vi "ReadMJPEGStream.vi"(11 "url":string="http://localhost:8000") -> (0 "error out":errorcluster, 2 "Info":T1, 3 "TCP out":refnum<k5>)   [LabVIEW 2020]
panel:
  out "path":string
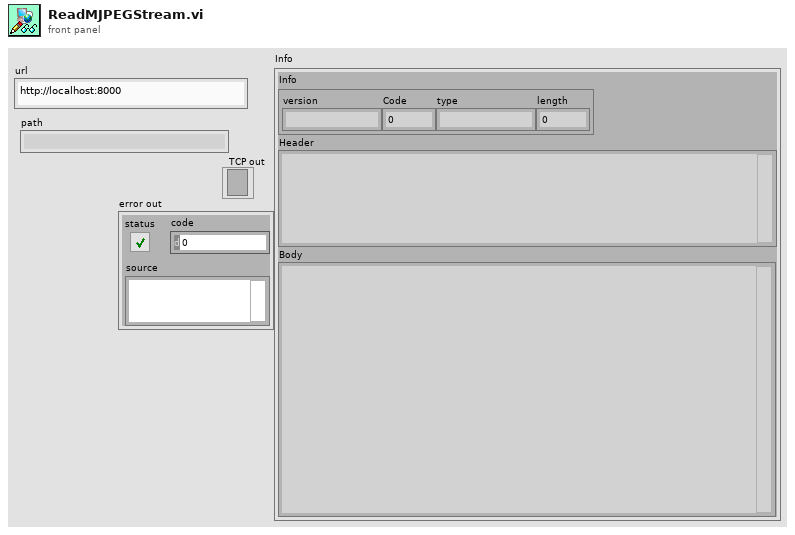
[diagram p1: front panel]
types:
  T1 = cluster{"Info":cluster{"version":string, "Code":i32, "type":string, "length":i32}, "Header":string, "Body":string}
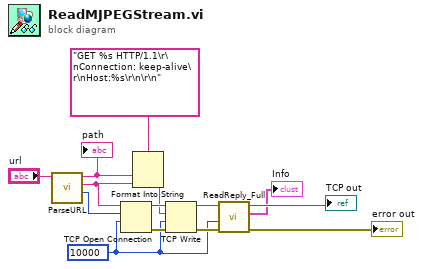
[diagram p0: block diagram]
diagram:
  w7 = 10000 ("timeout ms (60000)")
  n1 = call "ParseURL.vi"("url"="url") -> ("port"=w5:i32, "base url"=w4:string, "path"=w3:string)  [unwired: 8 in]
  "path" <- w3
  n2 = TCP Open Connection(address=w4, remote port or service name=w5, timeout ms (60000)=w7) -> (connection ID=w14:refnum<k5>, error out=w12:errorcluster)  [unwired: 2 in]
  n3 = Format Into String(format string="GET %s HTTP/1.1\r\nConnection: keep-alive\r\nHost:%s\r\n\r\n", w3, w4) -> (resulting string=w13:string)  [unwired: 2 in, 1 out]
  n4 = TCP Write(connection ID=w14, data in=w13, error in (no error)=w12, 9:w7) -> (connection ID out=w10:refnum<k5>, error out=w11:errorcluster)  [unwired: 1 out]
  n5 = call "ReadReply_Full.vi"("error in (no error)"=w11, "timeout ms (60000)"=w7, "TCP in"=w10) -> ("error out"=→"error out":errorcluster, "Info"=→"Info":T1, "TCP out"=→"TCP out":refnum<k5>)  [unwired: 6 in]
